vi "RT Main_EVO_V1_no_spike_text_file.vi"() -> ()   [LabVIEW 2017]
doc: "This template is for the Queued Message Handler design pattern.\n\nThe Event Handling Loop generates messages based on user interface actions.\n\nThe Message Handling Loop processes messages generated by the Event Handling Loop, or by other messages. The messages are string values, so new messages can be added easily to the Message Cases case structure in the Message Handling Loop. Each message cluster can also provide an optional value for Message Data, which is a variant that can be converted to whatever message-specific data is required."
uses:
  controls/FPGA State.ctl
  controls/Chatter data.ctl
  Globals/Global - All RT Loop Stop.vi
  <vilib>/rvi/errors/niLvFpgaAdjustHostInterfaceError.vi
  Globals/Global - Configuration Options.vi
  Globals/Global - RT Stream Connections.vi
  <vilib>/rvi/interface/nirviReadWriteControl/nirviReadWriteControl.xnode
  UI Error Handlers/support/Message Queue/Message Queue.lvlib
  NiFpgaLv.dll
  <vilib>/rvi/interface/Simulation/niFpgaSimulationCallBeginRW.vi
  <vilib>/nisyscfg/nisyscfg.lvlib
panel:
  out "Free Physical Memory or Largest Contiguous Memory (bytes)":i64(graph)
  in  "stop":bool
  out "G1 status":cluster{"G1 ":bool}
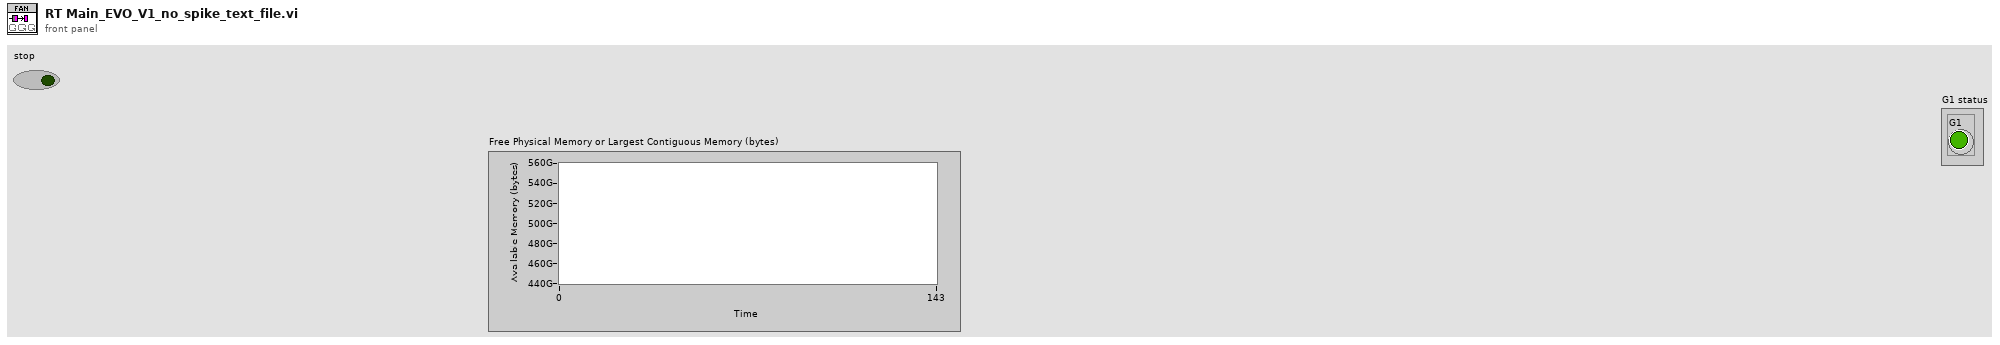
[diagram p1: front panel]
types:
  T1 = enum16{"open", "replace", "create", "open or create", "replace or create", "replace or create with confirmation"}
  T2 = typedef "Acceleration RT FIFO Reference.ctl" = refnum<k33>
  T3 = typedef "FPGA State.ctl" = enum16{"Safe State", "Control (PID)"}
  T4 = typedef "Chatter data.ctl" = cluster{"Tool data":cluster{"Number of teeth":sgl}, "Cutting data":cluster{"rpm":sgl}, "Limits":cluster{"Magnitude threshold":sgl, "Tolerance":sgl}, "G1 status":cluster{"G1 ":bool}}
  T5 = cluster{"FPGA State":T3, "Max Acceleration Threshold":sgl, "Chatter Data":T4}
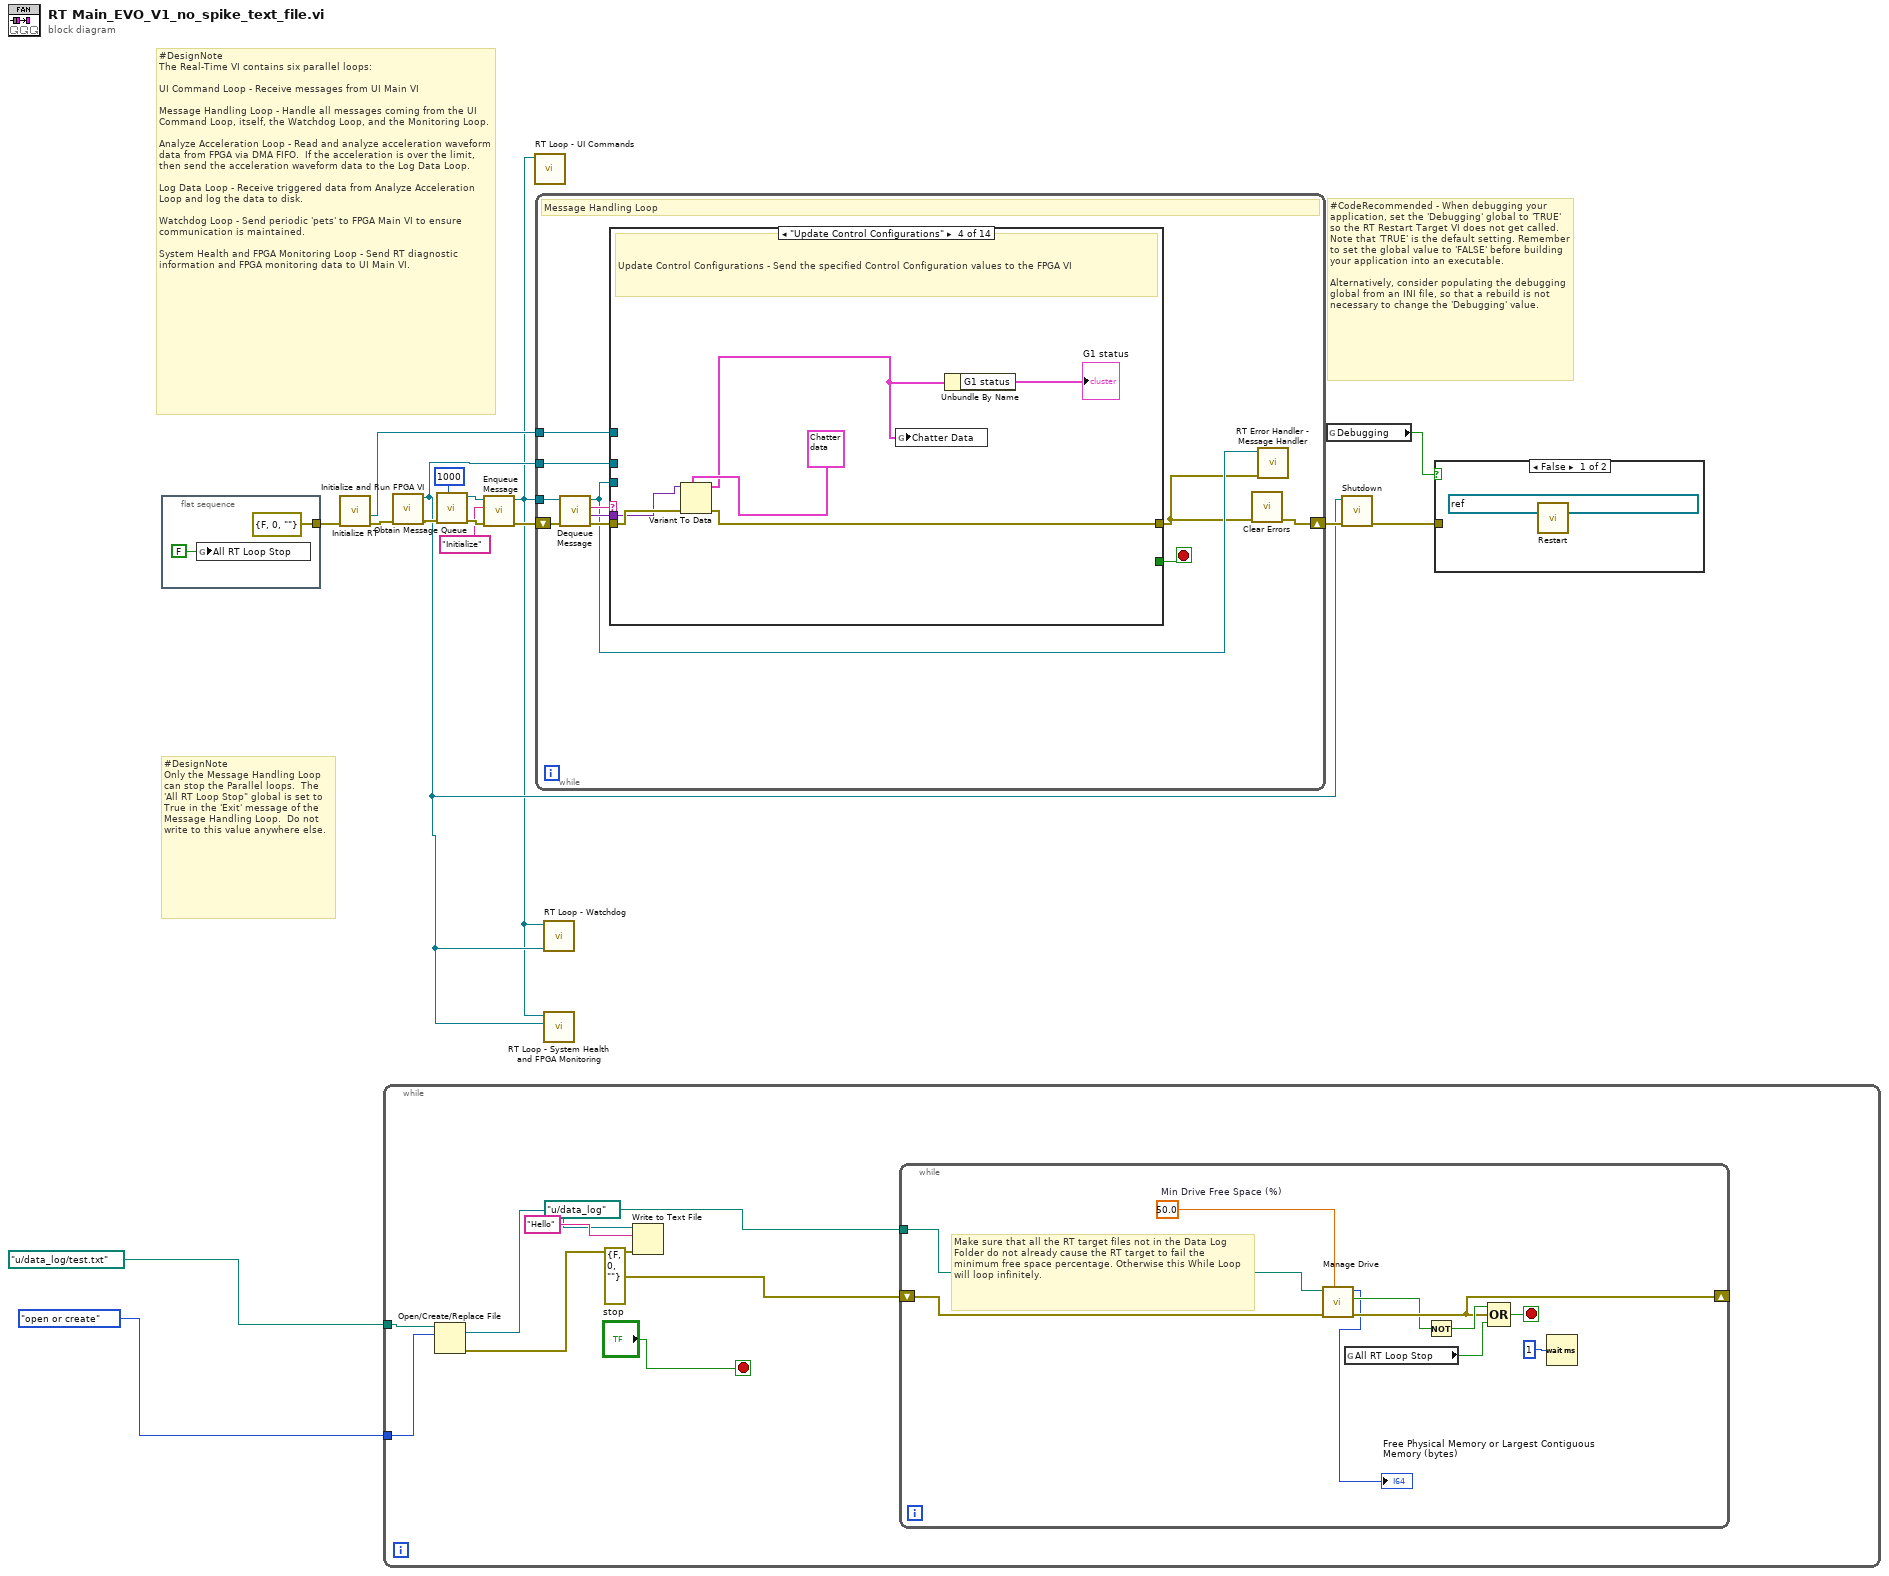
[diagram p0: block diagram]
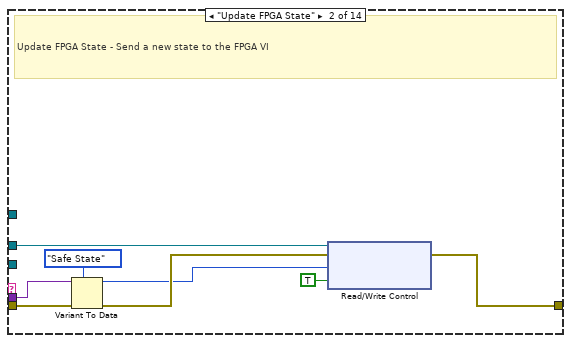
[diagram p4: hidden frame]
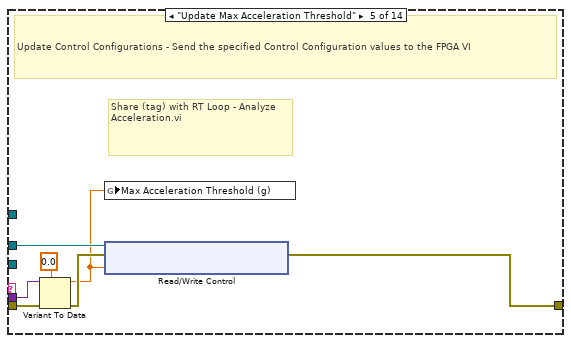
[diagram p6: hidden frame]
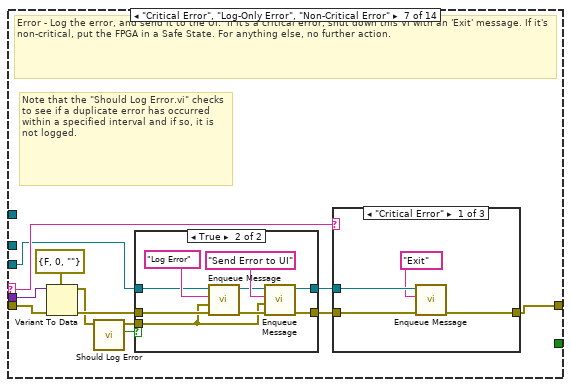
[diagram p8: hidden frame]
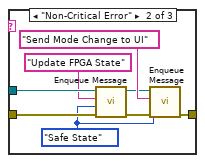
[diagram p10: hidden frame]
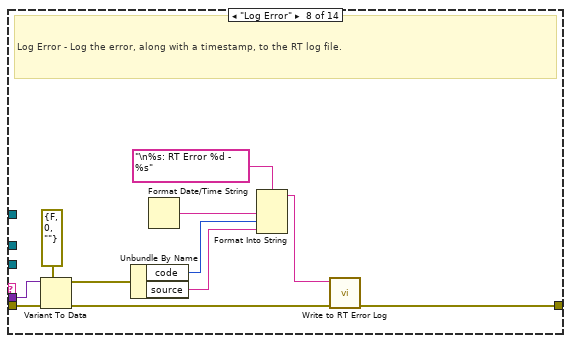
[diagram p12: hidden frame]
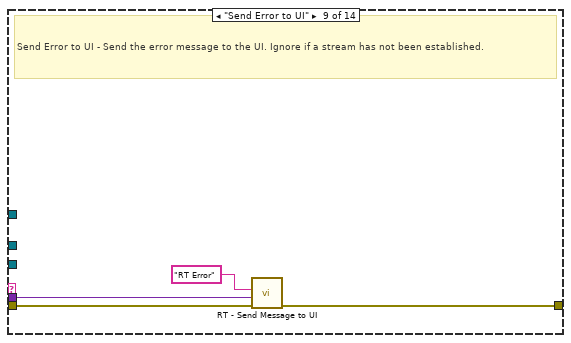
[diagram p13: hidden frame]
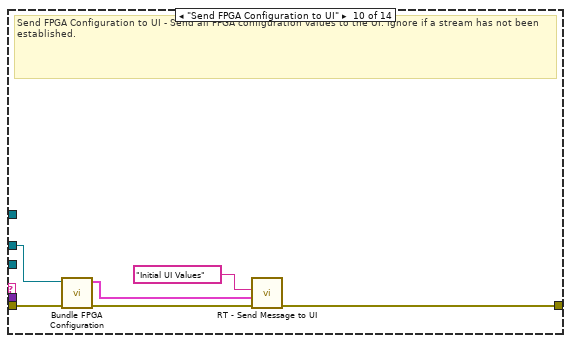
[diagram p14: hidden frame]
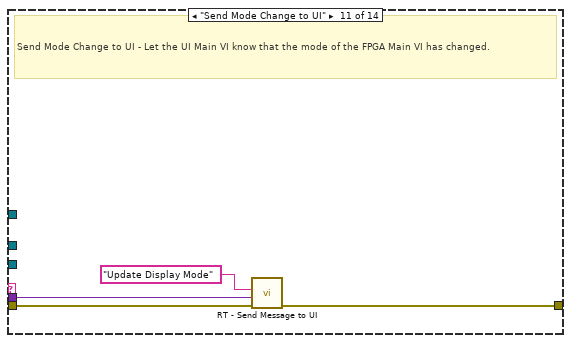
[diagram p15: hidden frame]
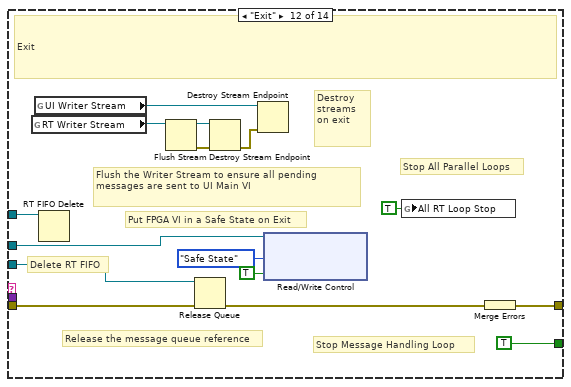
[diagram p16: hidden frame]
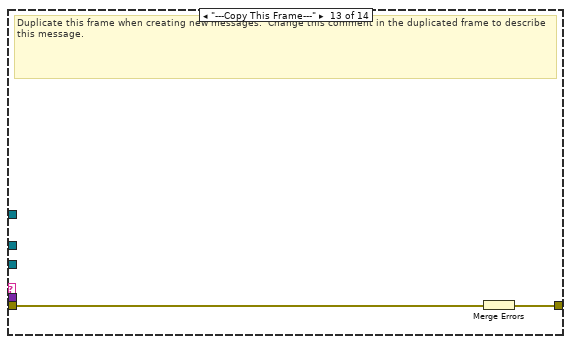
[diagram p17: hidden frame]
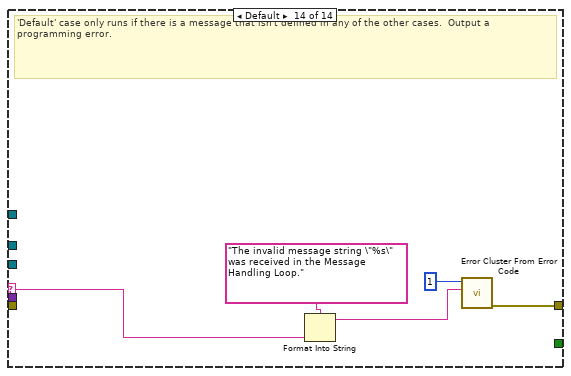
[diagram p18: hidden frame]
diagram:
  # "#CodeRecommended - When debugging your application, set the 'Debugging' global to 'TRUE' so the RT Restart Target VI does not get called.  Note that 'TRUE' is the default setting. Remember to set the global value to 'FALSE' before building your application into an executable.\n\nAlternatively, consider populating the debugging global from an INI file, so that a rebuild is not necessary to change the 'Debugging' value."
  # "#DesignNote\nThe Real-Time VI contains six parallel loops:\n\nUI Command Loop - Receive messages from UI Main VI\n\nMessage Handling Loop - Handle all messages coming from the UI Command Loop, itself, the Watchdog Loop, and the Monitoring Loop.\n\nAnalyze Acceleration Loop - Read and analyze acceleration waveform data from FPGA via DMA FIFO.  If the acceleration is over the limit, then send the acceleration waveform data to the Log Data Loop.\n\nLog Data Loop - Receive triggered data from Analyze Acceleration Loop and log the data to disk.\n\nWatchdog Loop - Send periodic 'pets' to FPGA Main VI to ensure communication is maintained.\n\nSystem Health and FPGA Monitoring Loop - Send RT diagnostic information and FPGA monitoring data to UI Main VI."
  # "#DesignNote\nOnly the Message Handling Loop can stop the Parallel loops.  The 'All RT Loop Stop\" global is set to True in the 'Exit' message of the Message Handling Loop.  Do not write to this value anywhere else."
  n1 = flat-sequence {
    tunnel: [errorcluster {"status"=FALSE, "code"=0, "source"=""} ("error constant")] -> w8
    frame #0 {
      n2 = global write "Global - All RT Loop Stop.vi" "All RT Loop Stop"(FALSE) -> ()
    }
  }
  n3 = call "Initialize RT.vi"("error in"=w8) -> ("error out"=w9:errorcluster, "Acceleration RT FIFO"=w5:T2)  [unwired: 8 in, 1 out]
  n4 = while {
    tunnel: T1."open or create" ("operation (0:open)") -> [w20]
    tunnel: path "u:/data_log/test.txt" ("file path (use dialog)") -> [w19]
    stop <- "stop" stop-if-true
    n5 = Open/Create/Replace File(file path (use dialog)=w19, operation (0:open)=w20) -> (refnum out=w21:refnum<file>, error out=w22:errorcluster)  [unwired: 4 in, 1 out]
    n6 = Write to Text File(file (use dialog)=w21, text="Hello", error in=w22) -> ()  [unwired: 1 in, 3 out]
    n7 = while {
      shift-right: [w31] -> _
      shift-left: errorcluster {"status"=FALSE, "code"=0, "source"=""} ("error out") -> [w32]
      tunnel: path "u:/data_log" ("AVI Path") -> [w29]
      stop <- w36 stop-if-true
      w30 = 50.0  # Min Drive Free Space (%)
      # "Make sure that all the RT target files not in the Data Log Folder do not already cause the RT target to fail the minimum free space percentage. Otherwise this While Loop will loop infinitely."
      n8 = call "Manage Drive.vi"("Min Drive Free Space (%)"=w30, "error in"=w32, "Data Folder"=w29) -> ("error out"=w31:errorcluster, "Drive Space Below Limit"=w28:bool, "size (bytes)"=→"Free Physical Memory or Largest Contiguous Memory (bytes)":i64)  [unwired: 6 in]
      n9 = global read "Global - All RT Loop Stop.vi" "All RT Loop Stop"() -> (w33:bool)
      n10 = Not(x=w28) -> (.not. x?=w35:bool)
      n11 = Compound Arithmetic op=OR(w35, w31, w33) -> (w36:bool)
      n12 = Wait (ms)(milliseconds to wait=u32 1) -> ()  [unwired: 1 out]
    }
  }
  n13 = call "Initialize and Run FPGA VI.vi"("error in (no error)"=w9) -> ("error out"=w12:errorcluster, "FPGA VI Reference Out 2"=w4:refnum<k20>)  [unwired: 9 in]
  n14 = call "Obtain Message Queue.vi"("max queue size (-1, unlimited)"=1000, "error in (no error)"=w12) -> ("error out"=w16:errorcluster, "Message Queue"=w15:refnum<queue>)  [unwired: 8 in]
  n15 = call "Enqueue Message.vi"("error in (no error)"=w16, "Message"="Initialize", "Message Queue"=w15) -> ("error out"=w13:errorcluster, "dup Message Queue"=w3:refnum<queue>)  [unwired: 7 in]
  n16 = call "RT Loop - UI Commands.vi"("Message Queue"=w3) -> ()  [unwired: 11 in]
  n17 = while {
    tunnel: w3 -> [w42]
    shift-right: [w39] -> w7
    shift-left: w13 -> [w46]
    tunnel: w4 -> [w41]
    tunnel: w5 -> [w37]
    stop <- w47 stop-if-true
    # "Message Handling Loop"
    n18 = call "Dequeue Message.vi"("error in (no error)"=w46, "Message Queue"=w42) -> ("error out"=w45:errorcluster, "Message Data"=w43:variant, "Message"=w44:string, "dup Message Queue"=w40:refnum<queue>)  [unwired: 6 in]
    n19 = case "Message Cases" shown="\"Update Control Configurations\"" w44 {
      selector: w44 -> [_ _ _ _ _ _ w81 _ _ _ _ _ _ w153]
      tunnel: w40 -> [_ _ _ _ _ _ w75 _ _ _ _ w147 _ _]
      tunnel: w45 -> [w48 w56 w57 w63 w70 w71 w79 w118 w122 w128 w132 w143 w149 _]
      tunnel: [w48 w53 w57 w62 w64 w71 w80 w109 w119 w125 w131 w144 w148 w151] -> w38
      tunnel: [_ _ _ _ _ _ _ _ _ _ _ TRUE _ _] -> w47
      tunnel: w43 -> [_ w55 _ w61 w69 _ w78 w117 w121 _ w130 _ _ _]
      tunnel: w41 -> [_ w51 _ _ w67 _ _ _ _ w124 _ w139 _ _]
      tunnel: w37 -> [_ _ _ _ _ _ _ _ _ _ _ w133 _ _]
      frame "Initialize" {
        # "Initialize - Currently a no-op for the RT Main VI"
      }
      frame "Update FPGA State" {
        # "Update FPGA State - Send a new state to the FPGA VI"
        n20 = Variant To Data(error in=w56, type=FPGA_State."Safe State" ("FPGA State"), Variant=w55) -> (data=w50:T3, error out=w52:errorcluster)
        n21 = xnode "Read/Write Control"("FPGA VI Reference In"=w51, "error in"=w52, "New FPGA State"=w50, "Change State"=TRUE) -> ("error out"=w53:errorcluster)  [unwired: 1 out]
      }
      frame "Update Setpoints" {
        # "Update Setpoints - Send the specified setpoint values to the FPGA VI"
      }
      frame "Update Control Configurations" {
        # "Update Control Configurations - Send the specified Control Configuration values to the FPGA VI"
        n22 = Variant To Data(error in=w63, type=T4 {"Tool data"={"Number of teeth"=2.0}, "Cutting data"={"rpm"=9898.0}, "Limits"={"Magnitude threshold"=0.0, "Tolerance"=1.0}, "G1 status"={"G1 "=FALSE}} ("Chatter Data"), Variant=w61) -> (data=w59:T4, error out=w62:errorcluster)
        n23 = global write "Global - Configuration Options.vi" "Chatter Data"(w59) -> ()
        n24 = Unbundle By Name(w59) -> ("G1 status"=→"G1 status":cluster{"G1 ":bool})
      }
      frame "Update Max Acceleration Threshold" {
        # "Share (tag) with RT Loop - Analyze Acceleration.vi"
        # "Update Control Configurations - Send the specified Control Configuration values to the FPGA VI"
        n25 = Variant To Data(error in=w70, type=sgl 0.0 ("SGL"), Variant=w69) -> (data=w65:sgl, error out=w68:errorcluster)
        n26 = global write "Global - Configuration Options.vi" "Max Acceleration Threshold (g)"(w65) -> ()
        n27 = xnode "Read/Write Control"("FPGA VI Reference In"=w67, "error in"=w68, "Max Acceleration Threshold (g)"=w65) -> ("error out"=w64:errorcluster)  [unwired: 1 out]
      }
      frame "Update Max Fan Speed Threshold" {
        # "Update Control Configurations - Send the specified Control Configuration values to the FPGA VI"
      }
      frame "Critical Error", "Log-Only Error", "Non-Critical Error" {
        # "Note that the \"Should Log Error.vi\" checks to see if a duplicate error has occurred within a specified interval and if so, it is not logged."
        # "Error - Log the error, and send it to the UI.  If it's a critical error, shut down this VI with an 'Exit' message. If it's non-critical, put the FPGA in a Safe State. For anything else, no further action."
        n28 = Variant To Data(error in=w79, type=errorcluster {"status"=FALSE, "code"=0, "source"=""} ("error out"), Variant=w78) -> (data=w73:errorcluster, error out=w76:errorcluster)
        n29 = call "Should Log Error.vi"("error to report"=w73) -> ("Should Log Error?"=w74:bool, "dup error to report"=w72:errorcluster)  [unwired: 9 in]
        n30 = case shown="True" w74 {
          tunnel: [w85 w92] -> w83
          tunnel: [w84 w91] -> w82
          tunnel: w75 -> [w84 w90]
          tunnel: w76 -> [w85 w87]
          tunnel: w72 -> [_ w86]
          frame False {
          }
          frame True {
            n31 = call "Enqueue Message.vi"("error in (no error)"=w87, "Message Data"=w86, "Message"="Log Error", "Message Queue"=w90) -> ("error out"=w88:errorcluster, "dup Message Queue"=w89:refnum<queue>)  [unwired: 6 in]
            n32 = call "Enqueue Message.vi"("error in (no error)"=w88, "Message Data"=w86, "Message"="Send Error to UI", "Message Queue"=w89) -> ("error out"=w92:errorcluster, "dup Message Queue"=w91:refnum<queue>)  [unwired: 6 in]
          }
        }
        n33 = case shown="\"Critical Error\"" w81 {
          tunnel: w83 -> [w98 w106 w107]
          tunnel: w82 -> [w96 w105 _]
          tunnel: [w97 w102 w107] -> w80
          frame "Critical Error" {
            n34 = call "Enqueue Message.vi"("error in (no error)"=w98, "Message"="Exit", "Message Queue"=w96) -> ("error out"=w97:errorcluster)  [unwired: 7 in, 1 out]
          }
          frame "Non-Critical Error" {
            w99 = FPGA_State."Safe State" ("FPGA State")
            n35 = call "Enqueue Message.vi"("error in (no error)"=w106, "Message Data"=w99, "Message"="Update FPGA State", "Message Queue"=w105) -> ("error out"=w103:errorcluster, "dup Message Queue"=w100:refnum<queue>)  [unwired: 6 in]
            n36 = call "Enqueue Message.vi"("error in (no error)"=w103, "Message Data"=w99, "Message"="Send Mode Change to UI", "Message Queue"=w100) -> ("error out"=w102:errorcluster)  [unwired: 6 in, 1 out]
          }
          frame Default {
          }
        }
      }
      frame "Log Error" {
        # "Log Error - Log the error, along with a timestamp, to the RT log file."
        n37 = Variant To Data(error in=w118, type=errorcluster {"status"=FALSE, "code"=0, "source"=""} ("error constant"), Variant=w117) -> (data=w112:errorcluster, error out=w115:errorcluster)
        n38 = Unbundle By Name(w112) -> ("code"=w111:i32, "source"=w110:string)
        n39 = Format Date/Time String() -> (date/time string=w113:string)  [unwired: 3 in]
        n40 = Format Into String(format string="\n%s: RT Error %d - %s", w113, w111, w110) -> (resulting string=w108:string)  [unwired: 2 in, 1 out]
        n41 = call "Write to RT Error Log.vi"("error in (no error)"=w115, "Log Entry"=w108) -> ("error out"=w109:errorcluster)  [unwired: 9 in]
      }
      frame "Send Error to UI" {
        # "Send Error to UI - Send the error message to the UI. Ignore if a stream has not been established."
        n42 = call "RT - Send Message to UI.vi"("error in (no error)"=w122, "Message Data"=w121, "Message"="RT Error") -> ("error out"=w119:errorcluster)  [unwired: 8 in]
      }
      frame "Send FPGA Configuration to UI" {
        # "Send FPGA Configuration to UI - Send all FPGA configuration values to the UI. Ignore if a stream has not been established."
        n43 = call "Bundle FPGA Configuration.vi"("error in (no error)"=w128, "FPGA VI Reference Out 2"=w124) -> ("error out"=w127:errorcluster, "Cluster"=w123:T5)  [unwired: 8 in]
        n44 = call "RT - Send Message to UI.vi"("error in (no error)"=w127, "Message Data"=w123, "Message"="Initial UI Values") -> ("error out"=w125:errorcluster)  [unwired: 8 in]
      }
      frame "Send Mode Change to UI" {
        # "Send Mode Change to UI - Let the UI Main VI know that the mode of the FPGA Main VI has changed."
        n45 = call "RT - Send Message to UI.vi"("error in (no error)"=w132, "Message Data"=w130, "Message"="Update Display Mode") -> ("error out"=w131:errorcluster)  [unwired: 8 in]
      }
      frame "Exit" {
        # "Delete RT FIFO"
        # "Flush the Writer Stream to ensure all pending messages are sent to UI Main VI"
        # "Destroy streams on exit"
        # "Put FPGA VI in a Safe State on Exit"
        # "Stop Message Handling Loop"
        # "Stop All Parallel Loops"
        # "Release the message queue reference"
        # "Exit"
        n46 = global read "Global - RT Stream Connections.vi" "RT Writer Stream"() -> (w136:refnum<k21>)
        n47 = global read "Global - RT Stream Connections.vi" "UI Writer Stream"() -> (w138:refnum<k21>)
        n48 = RT FIFO Delete(0:w133) -> ()  [unwired: 2 in, 1 out]
        n49 = Flush Stream(11:w136) -> (0:w134:errorcluster, 3:w135:refnum<k21>)  [unwired: 3 in, 1 out]
        n50 = Release Queue(queue=w147, error in (no error)=w143) -> (error out=w145:errorcluster)  [unwired: 1 in, 2 out]
        n51 = Destroy Stream Endpoint(8:w134, 11:w135) -> (0:w137:errorcluster)
        n52 = Destroy Stream Endpoint(8:w137, 11:w138) -> ()  [unwired: 1 out]
        n53 = xnode "Read/Write Control"("FPGA VI Reference In"=w139, "New FPGA State"=FPGA_State."Safe State" ("New State"), "Change State"=TRUE) -> ()  [unwired: 1 in, 2 out]
        n54 = global write "Global - All RT Loop Stop.vi" "All RT Loop Stop"(TRUE ("Stop Monitoring Loops")) -> ()
        n55 = Merge Errors(w145) -> (w144:errorcluster)
      }
      frame "---Copy This Frame---" {
        # "Duplicate this frame when creating new messages.  Change this comment in the duplicated frame to describe this message."
        n56 = Merge Errors(w149) -> (w148:errorcluster)
      }
      frame Default {
        # "'Default' case only runs if there is a message that isn't defined in any of the other cases.  Output a programming error."
        n57 = Format Into String(format string="The invalid message string \"%s\" was received in the Message Handling Loop." ("Unknown Message Error Text"), w153) -> (resulting string=w150:string)  [unwired: 2 in, 1 out]
        n58 = call <vilib>:"Error Cluster From Error Code.vi"("error message (\"\")"=w150, "error code (0)"=1) -> ("error out"=w151:errorcluster)  [unwired: 7 in]
      }
    }
    n59 = call <vilib>:"Clear Errors.vi"("error in (no error)"=w38) -> ("error out"=w39:errorcluster)  [unwired: 5 in, 1 out]
    n60 = call "RT Error Handler - Message Handler.vi"("error in (no error)"=w38, "Message Queue"=w40) -> ()  [unwired: 9 in, 1 out]
  }
  n61 = call "RT Loop - Watchdog.vi"("FPGA VI Reference in"=w4, "Message Queue"=w3) -> ()  [unwired: 10 in]
  n62 = call "RT Loop - System Health and FPGA Monitoring.vi"("FPGA VI Reference Out 2"=w4, "Message Queue"=w3) -> ()  [unwired: 9 in, 1 out]
  n63 = global read "Global - Configuration Options.vi" "Debugging"() -> (w11:bool)
  n64 = call "Shutdown.vi"("error in"=w7, "FPGA VI Reference in"=w4) -> ("error out"=w6:errorcluster)  [unwired: 9 in]
  n65 = case shown="False" w11 {
    tunnel: w6 -> [_ _]
    frame False {
      n66 = call <vilib>:"Restart.vi"("Session in"=refnum<k21> "NI-cRIO-9045-01DAA691 (143.167.159.188)" ("session in")) -> ()  [unwired: 8 in, 3 out]
    }
    frame True {
    }
  }
